vi "NearestPointAlgorithm.vi"(0 "Xref":dbl[](array[numeric]), 1 "Yref":dbl[](array[numeric]), 2 "Psiref":dbl[](array[numeric]), 3 "X estimate":dbl, 4 "Y estimate":dbl, 5 "Psi estimate":dbl, 6 "error in (no error)":errorcluster) -> (14 "error out":errorcluster)   [LabVIEW 2019]
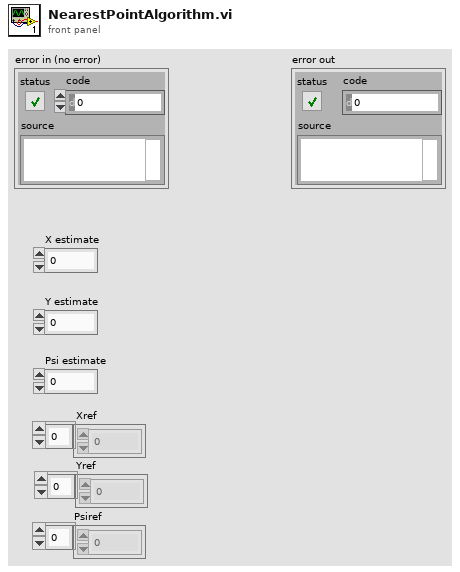
[diagram p1: front panel]
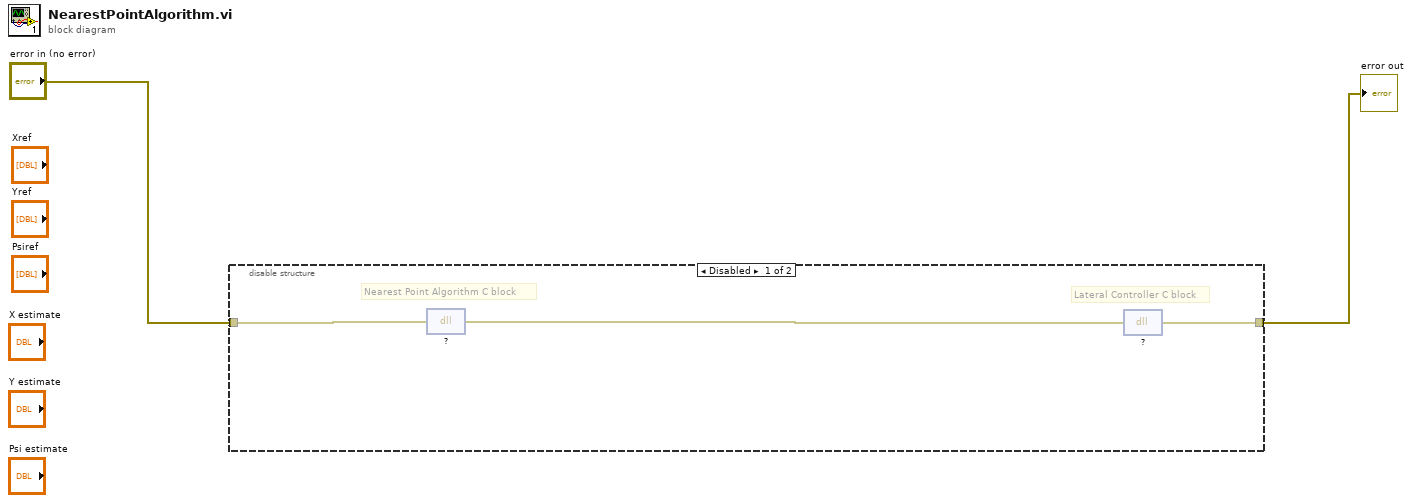
[diagram p0: block diagram]
diagram:
  n1 = disable-structure shown="Disabled" {
    disable-tunnel: "error in (no error)" -> [w5 _]
    disable-tunnel: [w3 _] -> w1
    frame Disabled {
      # "Lateral Controller C block"
      # "Nearest Point Algorithm C block"
      n2 = dll-call lib="?" fn="?"(error in=w5) -> (error out=w4:errorcluster)  [unwired: 3 in, 1 out]
      n3 = dll-call lib="?" fn="?"(error in=w4) -> (error out=w3:errorcluster)  [unwired: 3 in, 1 out]
    }
    frame Enabled {
    }
  }
  "error out" <- w1
